vi "phi_d.vi"(2 "error in (no error)":errorcluster, 3 "x_d":T1) -> (0 "error out":errorcluster, 1 "phi_d":T1)   [LabVIEW 2021]
uses:
  <vilib>/Analysis/Matrix/Datatypes/RealMatrix.ctl
  <vilib>/Analysis/Matrix/NI_Matrix.lvlib
panel:
  out "x":dbl
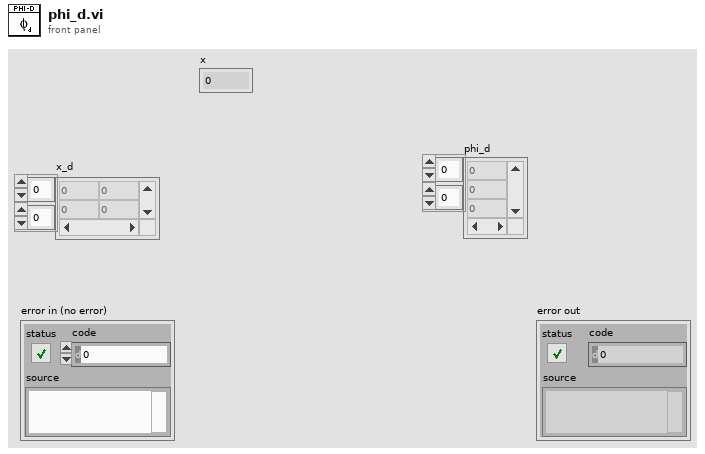
[diagram p1: front panel]
types:
  T1 = typedef "NI_Matrix.lvlib/RealMatrix.ctl" = dbl[][]
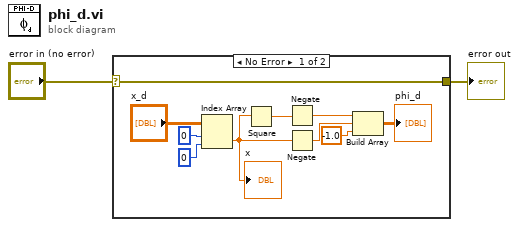
[diagram p0: block diagram]
diagram:
  n1 = case shown="No Error" "error in (no error)" {
    selector: "error in (no error)" -> [w4 w13]
    tunnel: [w4 w13] -> w1
    frame No Error {
      n2 = Index Array(array="x_d", index (row)=0, index (col)=0) -> (element=w5:dbl)
      "x" <- w5
      n3 = Square(x=w5) -> (x^2=w7:dbl)
      n4 = Negate(x=w7) -> (-x=w6:dbl)
      n5 = Negate(x=w5) -> (-x=w9:dbl)
      n6 = Build Array(w6, w9, -1.0) -> (→"phi_d":T1)
    }
    frame Error {
    }
  }
  "error out" <- w1
